vi "tb_acquisition_simio.vi"() -> ()   [LabVIEW 2011]
uses:
  <vilib>/Platform/TimedLoop/XDataNode/XDataNode.xnode
  <vilib>/Platform/TimedLoop/XDataNode/nitl_modes.ctl
  <vilib>/Platform/TimedLoop/XDataNode/XDNodeRunTimeDep.lvlib
  <vilib>/Platform/TimedLoop/XDataNode/wakeup.ctl
  <vilib>/Platform/TimedLoop/XDataNode/timing_clust.ctl
  <vilib>/eio/EIONode/EIONode.xnode
  <vilib>/rvi/DataTransferAndStorage/Container/XNode/niFpgaContainer.xnode
  <vilib>/rvi/FIFO/Fifo_Resource/nirvififoEmulationRead.vi
  <vilib>/rvi/FIFO/Fifo_Resource/nirvififoEmulationWrite.vi
panel:
  out "Waveform Chart":i16(graph)
  out "Numeric":i32
  out "acq timed out?":bool
  out "Data":u32[](array[numeric])
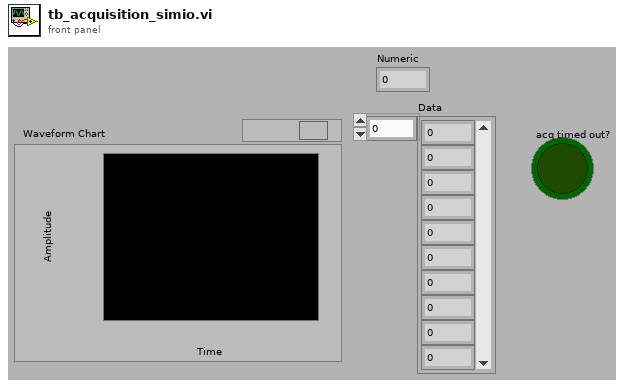
[diagram p1: front panel]
types:
  T1 = typedef "XDNodeRunTimeDep.lvlib/timing_clust.ctl" = cluster{"Expected End [f-1]":u64, "Actual End [f-1]":u64, "Finished Late? [f-1]":bool, "Expected End [i-1]":u64, "Actual End [i-1]":u64, "Finished Late? [i-1]":bool, "Expected Start [i]":u64, "Actual Start [i]":u64, "Expected Start [f]":u64, "Actual Start [f]":u64, "Source Name":string, "Structure Name":string, "Period":i64, "Deadline":i64, "Offset":i64, "Start":i64, "Priority":i32, "Timeout":i32, "Mode":T2, "Wakeup Reason":T3, "Error":errorcluster, "Source Type":string, "Secondary Source Type":string, "Global End Time":u64, "Global Start Time":u64, "Frame Duration":u64, "Iteration Duration":u64, "Assigned CPU":i32, "I/O Scan Engine Mode":u32}
  T2 = typedef "XDNodeRunTimeDep.lvlib/nitl_modes.ctl" = enum32{"No Change", "Process missed periods, maintain original phase", "Discard missed periods, maintain original phase", "Process missed periods, ignore original phase", "Discard missed periods, ignore original phase"}
  T3 = typedef "XDNodeRunTimeDep.lvlib/wakeup.ctl" = enum32{"Normal", "Aborted", "Asynchronous wakeup", "Timing source error", "Timed loop error", "Timeout"}
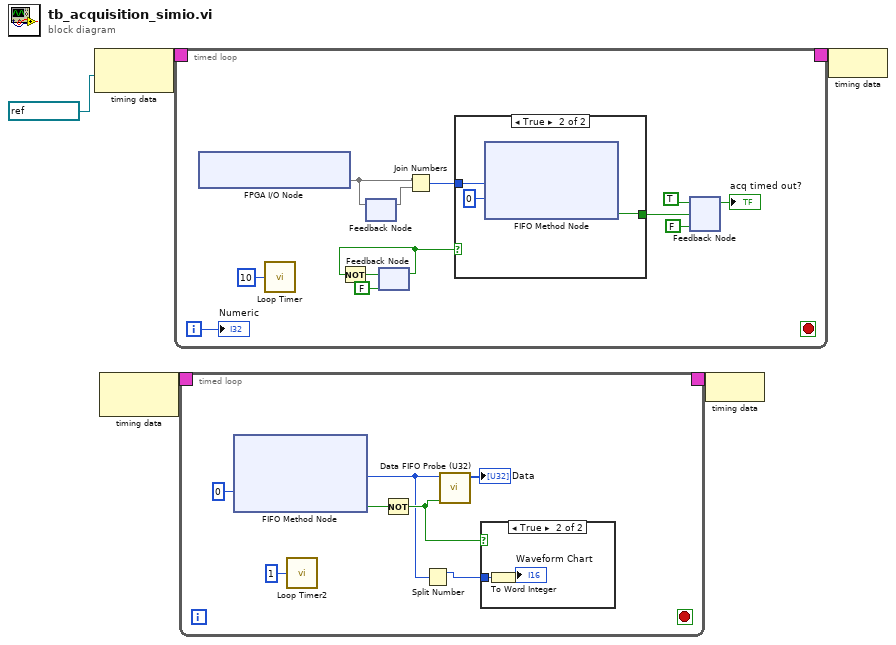
[diagram p0: block diagram]
diagram:
  n1 = node-c288(refnum<k21> "250MHz" ("Source Name")) -> (w5:T1)
  n2 = node-c288() -> (w2:T1)  [unwired: 1 in]
  n3 = timed-loop {
    timing: w5 -> [_]
    timing-out: [_] -> w4
    i -> [w8]
    stop <- _ stop-if-true
    n4 = xnode "FPGA I/O Node"() -> ("IO Module\\AI 0 Data"=w17)  [unwired: 1 in, 1 out]
    n5 = call "Loop Timer"("Count(mSec)"=u32 10) -> ()  [unwired: 1 out]
    n6 = feedback-in #1(w17) -> ()
    n7 = feedback #1() -> (w16)  [unwired: 1 in]
    n8 = feedback #2(FALSE) -> (w7:bool)
    n9 = Not(x=w7) -> (.not. x?=w15:bool)
    n10 = feedback-in #2(w15) -> ()
    n11 = Join Numbers(hi=w17, lo=w16) -> ((hi.lo)=w6:u32)
    n12 = case shown="True" w7 {
      tunnel: w6 -> [_ w20]
      tunnel: [_ w18] -> w11
      frame False {
      }
      frame True {
        n13 = xnode ("FIFO Method Node")("Element"=w20, "Timeout"=0) -> ("Timed Out?"=w18:bool)  [unwired: 1 in, 1 out]
      }
    }
    n14 = feedback-in #3(TRUE, w11) -> ()
    n15 = feedback #3(FALSE) -> (→"acq timed out?":bool)
    "Numeric" <- w8
  }
  n16 = timed-loop {
    timing: w2 -> [_]
    timing-out: [_] -> w1
    stop <- _ stop-if-true
    n17 = xnode ("FIFO Method Node")("Timeout"=0) -> ("Element"=w24:u32, "Timed Out?"=w28:bool)  [unwired: 1 in, 1 out]
    n18 = call "Loop Timer2"("Count(mSec)"=u32 1) -> ()  [unwired: 1 out]
    n19 = Not(x=w28) -> (.not. x?=w25:bool)
    n20 = Split Number(x=w24) -> (hi(x)=w23:u16)  [unwired: 1 out]
    n21 = call <userlib>:"Data FIFO Probe (U32).vi"("Valid"=w25, "Data"=w24) -> ("Array"=→"Data":u32[])  [unwired: 9 in]
    n22 = case shown="True" w25 {
      tunnel: w23 -> [_ w31]
      frame False {
      }
      frame True {
        n23 = To Word Integer(number=w31) -> (16bit integer=→"Waveform Chart":i16)
      }
    }
  }
  n24 = node-c288(w1) -> ()
  n25 = node-c288(w4) -> ()
